vi "z string array clone.vi"(8 "error in (no error)":errorcluster, 10 "this_":cluster{}, 11 "dst":cluster{}) -> (0 "error out":errorcluster, 3 "dst out":cluster{})   [LabVIEW 2021, in "zenohc.lvlib"]
doc: "void z_string_array_clone(struct z_owned_string_array_t *dst,\n const struct z_loaned_string_array_t *this_);"
uses:
  zenohc.lvlib
  zenohc.dll
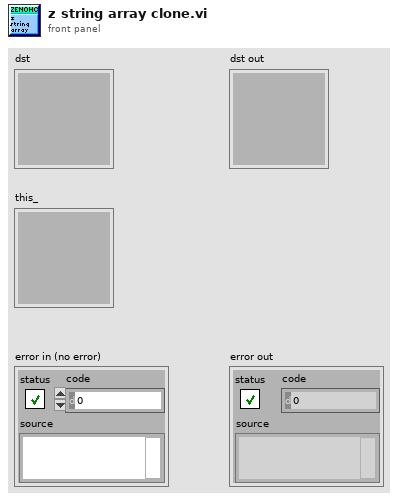
[diagram p1: front panel]
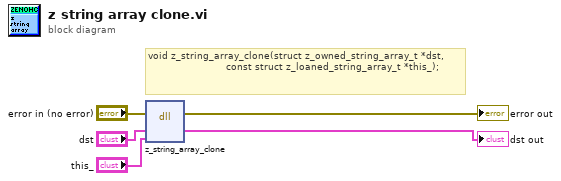
[diagram p0: block diagram]
diagram:
  # "void z_string_array_clone(struct z_owned_string_array_t *dst,\n                          const struct z_loaned_string_array_t *this_);"
  n1 = dll-call lib="D:/dev/zenoh_labview/zenohc/zenohc.*" fn="z_string_array_clone"(error in="error in (no error)", "dst"="dst", "this_"="this_") -> (error out=→"error out":errorcluster, "dst"=→"dst out":cluster{})  [unwired: 4 in, 1 out]
